vi "test Value to String to Value (Numeric).vi"(8 "error in":errorcluster, 11 "TestCase in":refnum<class "SharedUtilities.lvclass">) -> (0 "error out":errorcluster, 3 "TestCase out":refnum<class "SharedUtilities.lvclass">)   [LabVIEW 2020, in "SharedUtilities.lvclass"]
uses:
  SharedUtilities.lvclass
  a84d69d1-fad3-47e2-8154-2ef23eda858b.vi
  632cccee-0c4c-48ba-a1a1-d530fae7511a.vi
  73afe90c-fb02-4216-b4a1-b923eed82594.vi
  028d73e9-00fb-4542-a23b-66b9e29aa0b1.vi
  498c05f8-15b5-4ac0-8c3d-e5ac85a5572c.vi
  9906eb62-703c-4add-a383-eb4992a64633.vi
  765adaa7-6db4-4e08-a474-63e678192e54.vi
  56418cb7-ba00-4197-a567-0162e8e05559.vi
  124e4a82-a322-4f77-b708-c9a9df3cc2a7.vi
  e176098c-f1c9-4183-b6cb-0c3193a36cca.vi
  be1d5e8e-978c-410b-8566-c301a53a3bbb.vi
  bffcf280-2935-4e02-95a8-f0f358590e1d.vi
  daa5d11f-5b99-42f1-8834-9841ad71a453.vi/a245c9b3-7860-4378-b45d-1a18453f9496.vi
  265a4f6a-8fc9-49a9-87da-2e0427092cad.vi/c48ddff9-9a8b-496e-9eda-6cc446fe6a52.vi
  604a061f-c667-495c-94b7-c918dc8a8267.vi/20554e8c-3db0-4abe-8101-32459e180398.vi
  bf69ac35-1538-4543-b1b8-e28ddb0a0dbf.vi/3da32636-cfcd-4dcf-a9c9-441aaebdc3f7.vi
  f59cd133-b754-4db2-8afd-bd5022b0e04c.vi/4a3d9d72-8bc0-4889-a65e-20aac6576b9a.vi
  ff14866a-8100-4de3-b7d9-e60e69b5ce48.vi/342115b9-8d84-4172-a6e3-b68297bcda7c.vi
  69746de9-d8b8-4851-ac61-6c07aaca97d1.vi/e370109e-7b1f-4723-95cd-a7f314fa3b66.vi
  ff55a742-3439-4801-888b-e49006c659a7.vi/f027e316-7ebe-4211-a908-52e146f38046.vi
  a53efd5e-1b89-4488-9cb0-ebdcaa892606.vi/897f128d-c55e-4925-aa9f-655ec4de68c8.vi
  e7dd0ea7-1b51-4b32-9c58-6851ae4c1315.vi/575036ce-1d77-4ed0-ba25-f1c2de4d931f.vi
  0f61251e-6bce-40bc-9127-ed727464e5d8.vi/fef4707d-1d88-4ef5-8383-a3ef5d137053.vi
  4657b86e-0f3a-47b0-a768-c094f0f21e47.vi/b0c5697e-586e-4791-862a-2ae83e906fde.vi
  <vilib>/addons/_JKI Toolkits/VI Tester/TestCase.llb/TestCase.lvclass
  C:/Program Files (x86)/National Instruments/LabVIEW 2020/vi.lib/addons/_JKI Toolkits/VI Tester/TestCase.llb/TestCase.lvclass
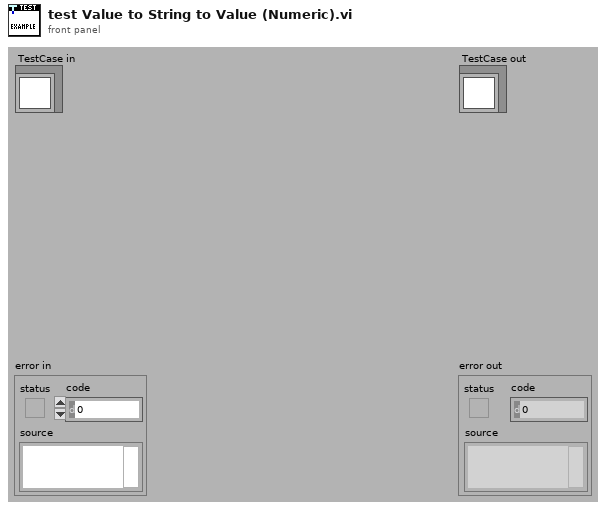
[diagram p1: front panel]
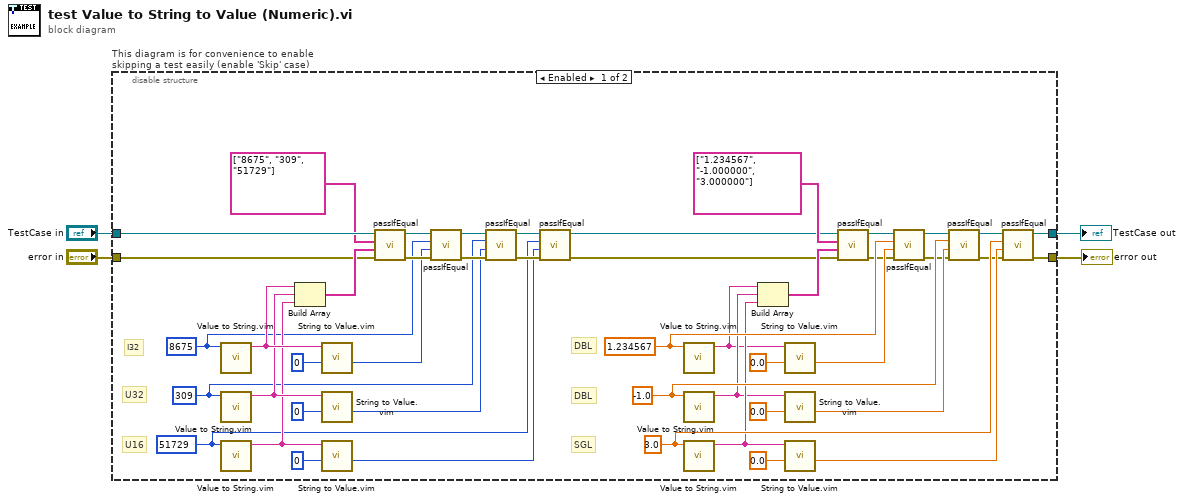
[diagram p0: block diagram]
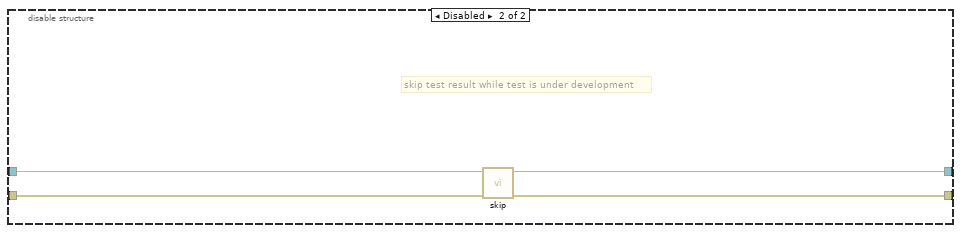
[diagram p2: hidden frame]
diagram:
  n1 = disable-structure "This diagram is for convenience to enable skipping a test easily (enable 'Skip' case)" shown="Enabled" {
    disable-tunnel: "TestCase in" -> [w50 w54]
    disable-tunnel: [w6 w52] -> w1
    disable-tunnel: [w5 w53] -> w3
    disable-tunnel: "error in" -> [w41 w51]
    frame Enabled {
      w27 = sgl 3.0
      w25 = -1.0
      w23 = 1.234567
      w30 = u16 51729
      w32 = u32 309
      w34 = 8675
      # "U16"
      # "U32"
      # "I32"
      # "SGL"
      # "DBL"
      # "DBL"
      n2 = call "Value to String.vim"("value"=w34) -> ("string"=w46:string)  [unwired: 10 in]
      n3 = call "Value to String.vim"("value"=w32) -> ("string"=w45:string)  [unwired: 10 in]
      n4 = call "Value to String.vim"("value"=w30) -> ("string"=w44:string)  [unwired: 10 in]
      n5 = Build Array(w46, w45, w44) -> (w43:string[])
      n6 = call "String to Value.vim"("default"=0, "string"=w46) -> ("value"=w33:i32)  [unwired: 9 in]
      n7 = call "String to Value.vim"("default"=u32 0, "string"=w45) -> ("value"=w31:u32)  [unwired: 9 in]
      n8 = call "String to Value.vim"("default"=u16 0, "string"=w44) -> ("value"=w29:u16)  [unwired: 9 in]
      n9 = call-dynamic "passIfEqual.vi"("error in (no error)"=w41, "y"=w43, "x"=string[] ["8675", "309", "51729"] ("appended array"), "TestCase in"=w50) -> ("error out"=w40:errorcluster, "TestCase out"=w39:refnum<class "SharedUtilities.lvclass">)  [unwired: 6 in]
      n10 = call-dynamic "passIfEqual.vi"("error in (no error)"=w40, "y"=w33, "x"=w34, "TestCase in"=w39) -> ("error out"=w38:errorcluster, "TestCase out"=w37:refnum<class "SharedUtilities.lvclass">)  [unwired: 6 in]
      n11 = call-dynamic "passIfEqual.vi"("error in (no error)"=w38, "y"=w31, "x"=w32, "TestCase in"=w37) -> ("error out"=w36:errorcluster, "TestCase out"=w35:refnum<class "SharedUtilities.lvclass">)  [unwired: 6 in]
      n12 = call-dynamic "passIfEqual.vi"("error in (no error)"=w36, "y"=w29, "x"=w30, "TestCase in"=w35) -> ("error out"=w7:errorcluster, "TestCase out"=w8:refnum<class "SharedUtilities.lvclass">)  [unwired: 6 in]
      n13 = call "Value to String.vim"("value"=w23) -> ("string"=w12:string)  [unwired: 10 in]
      n14 = call "Value to String.vim"("value"=w25) -> ("string"=w13:string)  [unwired: 10 in]
      n15 = call "Value to String.vim"("value"=w27) -> ("string"=w14:string)  [unwired: 10 in]
      n16 = Build Array(w12, w13, w14) -> (w15:string[])
      n17 = call "String to Value.vim"("default"=0.0, "string"=w12) -> ("value"=w24:dbl)  [unwired: 9 in]
      n18 = call "String to Value.vim"("default"=0.0, "string"=w13) -> ("value"=w26:dbl)  [unwired: 9 in]
      n19 = call "String to Value.vim"("default"=sgl 0.0, "string"=w14) -> ("value"=w28:sgl)  [unwired: 9 in]
      n20 = call-dynamic "passIfEqual.vi"("error in (no error)"=w7, "y"=w15, "x"=string[] ["1.234567", "-1.000000", "3.000000"] ("appended array"), "TestCase in"=w8) -> ("error out"=w17:errorcluster, "TestCase out"=w18:refnum<class "SharedUtilities.lvclass">)  [unwired: 6 in]
      n21 = call-dynamic "passIfEqual.vi"("error in (no error)"=w17, "y"=w24, "x"=w23, "TestCase in"=w18) -> ("error out"=w19:errorcluster, "TestCase out"=w20:refnum<class "SharedUtilities.lvclass">)  [unwired: 6 in]
      n22 = call-dynamic "passIfEqual.vi"("error in (no error)"=w19, "y"=w26, "x"=w25, "TestCase in"=w20) -> ("error out"=w21:errorcluster, "TestCase out"=w22:refnum<class "SharedUtilities.lvclass">)  [unwired: 6 in]
      n23 = call-dynamic "passIfEqual.vi"("error in (no error)"=w21, "y"=w28, "x"=w27, "TestCase in"=w22) -> ("error out"=w5:errorcluster, "TestCase out"=w6:refnum<class "SharedUtilities.lvclass">)  [unwired: 6 in]
    }
    frame Disabled {
      # "skip test result while test is under development"
      n24 = call <vilib>:"skip.vi"("error in (no error)"=w51, "TestCase in"=w54) -> ("error out"=w53:errorcluster, "TestCase out"=w52:refnum<class "SharedUtilities.lvclass">)  [unwired: 8 in]
    }
  }
  "error out" <- w3
  "TestCase out" <- w1
